vi "ADC esp-32 (SubVI).vi"(3 "error in (no error)":errorcluster, 5 "VISA Refnum in":refnum<visa-resource-name>="COM7") -> (0 "error out":errorcluster, 1 "value adc":i16, 2 "VISA resource name out":refnum<visa-resource-name>)   [LabVIEW 2018]
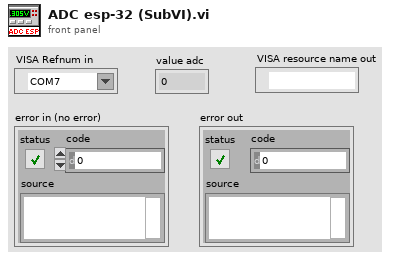
[diagram p1: front panel]
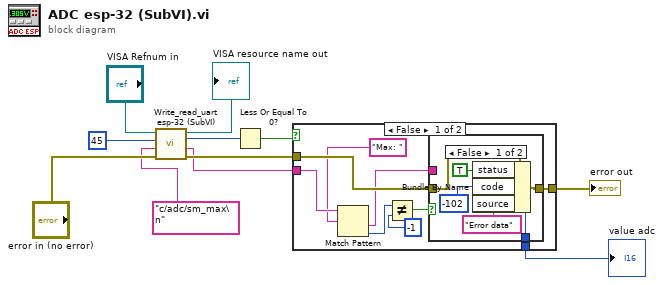
[diagram p0: block diagram]
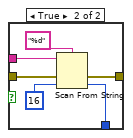
[diagram p2: hidden frame]
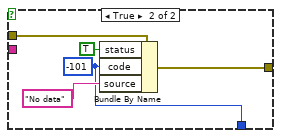
[diagram p3: hidden frame]
diagram:
  n1 = call "Write_read_uart esp-32 (SubVI).vi"("error in (no error)"="error in (no error)", "write buffer"="c/adc/sm_max\n", "milliseconds to wait"=u32 45, "VISA Refnum in"="VISA Refnum in") -> ("error out 4"=w4:errorcluster, "read buffer"=w2:string, "read bite"=w7:u32, "VISA resource name out"=→"VISA resource name out":refnum<visa-resource-name>)
  n2 = Less Or Equal To 0?(x=w7) -> (x <= 0?=w5:bool)
  n3 = case shown="False" w5 {
    tunnel: w4 -> [w20 w36]
    tunnel: [w19 w33] -> w3
    tunnel: w2 -> [w18 _]
    tunnel: [w12 w32] -> w1
    frame False {
      n4 = Match Pattern(string=w18, regular expression="Max: ") -> (after substring=w13:string, offset past match=w16:i32)  [unwired: 1 in, 2 out]
      n5 = Not Equal?(x=w16, y=-1 ("offset past match")) -> (x != y?=w14:bool)
      n6 = case shown="False" w14 {
        tunnel: w20 -> [w25 w31]
        tunnel: [w24 w30] -> w19
        tunnel: w13 -> [_ w27]
        tunnel: [w21 w26] -> w12
        frame False {
          w21 = i16 -102 ("code")
          n7 = Bundle By Name(cluster=w25, "status"=TRUE, "code"=w21, "source"="Error data") -> (w24:errorcluster)
        }
        frame True {
          n8 = Scan From String(format string="%d", input string=w27, error in=w31, default 1=i16 16 ("default value 1")) -> (error out=w30:errorcluster, output 1=w26:i16)  [unwired: 1 in, 2 out]
        }
      }
    }
    frame True {
      w32 = i16 -101 ("code")
      n9 = Bundle By Name(cluster=w36, "status"=TRUE, "code"=w32, "source"="No data") -> (w33:errorcluster)
    }
  }
  "error out" <- w3
  "value adc" <- w1
